vi "MOSES_v8.vi"(7 "Scan List (empty)":string="101:132,201:222", 8 "error in (no error)":errorcluster, 9 "Range (5:Auto)":T3(ring)=enum."Auto", 10 "Resolution (5:Default)":T2(ring)=enum."Default", 11 "VISA resource name":refnum<visa-resource-name>="GPIB0::9::INSTR") -> (0 "error out":errorcluster, 2 "Output Array":dbl[](array[numeric]) format="%.2f", 3 "VISA resource name out":refnum<visa-resource-name>)   [LabVIEW 2013]
doc: "This VI allows you to take simple voltage measurements from the instrument."
uses:
  Instance          12 13Saved   MOSES .vi
  Instance          62 13Saved   MOSES .vi
  Instance          11 13Saved   MOSES .vi
  Instance          63 13Saved   MOSES .vi
  Instance           9 13Saved   MOSES .vi
  Instance          64 13Saved   MOSES .vi
  Instance          10 13Saved   MOSES .vi
  Instance          60 13Saved   MOSES .vi
  Instance           8 13Saved   MOSES .vi
  Instance          33 13Saved   MOSES .vi
  Instance          75 13Saved   MOSES .vi
  Instance          37 13Saved   MOSES .vi
  Instance           5 13Saved   MOSES .vi
  Instance          32 13Saved   MOSES .vi
  Instance          74 13Saved   MOSES .vi
  Instance          38 13Saved   MOSES .vi
  Instance          72 13Saved   MOSES .vi
  Instance          41 13Saved   MOSES .vi
  Instance          71 13Saved   MOSES .vi
  Instance          40 13Saved   MOSES .vi
  Instance          73 13Saved   MOSES .vi
  Instance          39 13Saved   MOSES .vi
  Instance           6 13Saved   MOSES .vi
  Instance          35 13Saved   MOSES .vi
  Instance           7 13Saved   MOSES .vi
  Instance           4 13Saved   MOSES .vi
  Instance          34 13Saved   MOSES .vi
  Instance          16 13Saved   MOSES .vi
  Instance          52 13Saved   MOSES .vi
  Instance          17 13Saved   MOSES .vi
  Instance          58 13Saved   MOSES .vi
  Instance           1 13Saved   MOSES .vi
  Instance          53 13Saved   MOSES .vi
  Instance          15 13Saved   MOSES .vi
  Instance          59 13Saved   MOSES .vi
  Instance          19 13Saved   MOSES .vi
  Instance          57 13Saved   MOSES .vi
  Instance          18 13Saved   MOSES .vi
  Instance          56 13Saved   MOSES .vi
  Instance          20 13Saved   MOSES .vi
  Instance          55 13Saved   MOSES .vi
  Instance          22 13Saved   MOSES .vi
  Instance          54 13Saved   MOSES .vi
  Instance          21 13Saved   MOSES .vi
  Instance          51 13Saved   MOSES .vi
  Instance           2 13Saved   MOSES .vi
  Instance          50 13Saved   MOSES .vi
  Instance          23 13Saved   MOSES .vi
  Instance          49 13Saved   MOSES .vi
  Instance          24 13Saved   MOSES .vi
  Instance          48 13Saved   MOSES .vi
  Instance          26 13Saved   MOSES .vi
  Instance          47 13Saved   MOSES .vi
  Instance           3 13Saved   MOSES .vi
  Instance          70 13Saved   MOSES .vi
  Instance          27 13Saved   MOSES .vi
  Instance          66 13Saved   MOSES .vi
  Instance          25 13Saved   MOSES .vi
  Instance          69 13Saved   MOSES .vi
  Instance          28 13Saved   MOSES .vi
  Instance          68 13Saved   MOSES .vi
  Instance          30 13Saved   MOSES .vi
  Instance          67 13Saved   MOSES .vi
  Instance          31 13Saved   MOSES .vi
  Instance          45 13Saved   MOSES .vi
  Instance          29 13Saved   MOSES .vi
  Instance          44 13Saved   MOSES .vi
  Instance          65 13Saved   MOSES .vi
  Instance          43 13Saved   MOSES .vi
  Instance          46 13Saved   MOSES .vi
  Instance          42 13Saved   MOSES .vi
  Instance          36 13Saved   MOSES .vi
  Instance          13 13Saved   MOSES .vi
  Instance          14 13Saved   MOSES .vi
  Instance          61 13Saved   MOSES .vi
panel:
  in  "?":T1(tab)
  out "TEC L -y":dbl
  out "Battery":dbl
  out "Boolean 10":bool
  out "Boolean 11":bool
  out "Boolean 12":bool
  out "Mains from IS":dbl
  out "Boolean 13":bool
  out "Boolean 14":bool
  out "Boolean 15":bool
  out "12d+, MTR2812D Out":dbl
  out "Boolean 16":bool
  out "Boolean 17":bool
  out "5s, MGA2805S Out":dbl
  out "Boolean 26":bool
  out "Boolean 27":bool
  out "IS Out":dbl
  out "Boolean 20":bool
  out "Boolean 21":bool
  out "Boolean 22":bool
  out "12d+ MTR2812D Out":dbl
  out "Boolean 23":bool
  out "Boolean 24":bool
  out "Boolean 25":bool
  out "5s MGA2805S Out":dbl
  out "Boolean 29":bool
  out "Boolean 30":bool
  out "Boolean 31":bool
  out "Power Supply Filter Input":dbl
  out "Boolean 67":bool
  out "Boolean 68":bool
  out "Boolean 90":bool
  out "Boolean 7":bool
  out "Boolean 8":bool
  out "TEC L +y":dbl
  out "Boolean 6":bool
  out "Boolean 5":bool
  out "TEC L 0y":dbl
  out "Boolean 9":bool
  out "Boolean 18":bool
  out "TEC R +y":dbl
  out "Boolean 19":bool
  out "Boolean 45":bool
  out "TEC R -y":dbl
  out "Boolean 46":bool
  out "Boolean 75":bool
  out "TEC R 0y":dbl
  out "Boolean 76":bool
  out "Boolean 89":bool
  out "Thermal 5V power":dbl
  out "Shutter 28V power":dbl
  out "H-alpha filter":dbl
  out "H-alpha camera":dbl
  out "ROE power supply input":dbl
  out "Premod filter positive 12V input":dbl
  out "Premod filter 5V input":dbl
  out "Shutter 28V power":dbl
  out "H-alpha filter":dbl
  out "ROE power supply input":dbl
  out "Boolean 41":bool
  out "Boolean 42":bool
  out "Res +y":dbl
  out "Res -y":dbl
  out "Res Back":dbl
  out "Boolean 43":bool
  out "Boolean 44":bool
  out "Boolean 47":bool
  out "Boolean 48":bool
  out "Boolean 49":bool
  out "Boolean 50":bool
  out "CF +y":dbl
  out "CF -y":dbl
  out "CF 0y":dbl
  out "Boolean 51":bool
  out "Boolean 52":bool
  out "Boolean 53":bool
  out "Boolean 54":bool
  out "BP +y":dbl
  out "BP -y":dbl
  out "BP 0y":dbl
  out "Boolean 55":bool
  out "Boolean 56":bool
  out "Boolean 57":bool
  out "Boolean 58":bool
  out "Boolean 59":bool
  out "Boolean 60":bool
  out "Boolean 40":bool
  out "PCU Res":dbl
  out "Boolean 83":bool
  out "Boolean 84":bool
  out "ICU":dbl
  out "Boolean 85":bool
  out "Boolean 86":bool
  out "PCU Box":dbl
  out "Boolean 87":bool
  out "Boolean 88":bool
  out "Boolean 32":bool
  out "Boolean 33":bool
  out "Boolean 34":bool
  out "TEC +y":dbl
  out "TEC -y":dbl
  out "TEC 0y":dbl
  out "Boolean 35":bool
  out "Boolean 36":bool
  out "Boolean 37":bool
  out "Boolean 38":bool
  out "Boolean 39":bool
  out "Comp Res":dbl
  out "Boolean 61":bool
  out "Boolean 62":bool
  out "Vortec x86 CPU":dbl
  out "Boolean 63":bool
  out "Boolean 64":bool
  out "Mainboard":dbl
  out "Boolean 65":bool
  out "Boolean 66":bool
  out "Virtex 5 FPGA":dbl
  out "Boolean 69":bool
  out "Boolean 70":bool
  out "RPA":dbl
  out "Boolean 71":bool
  out "Boolean 72":bool
  out "TC Res.":dbl
  out "Boolean 73":bool
  out "Boolean 74":bool
  out "T CONT b -y":dbl
  out "Boolean 77":bool
  out "Boolean 78":bool
  out "12S":dbl
  out "Boolean 79":bool
  out "Boolean 80":bool
  out "12D":dbl
  out "Boolean 81":bool
  out "Boolean 82":bool
  out "0 Order TECs":dbl[][](graph)
  out "-1 Order TECs":dbl[][](graph)
  out "+1 Order TECs":dbl[][](graph)
  out "I5s":dbl[](graph)
  out "I12d+":dbl[](graph)
  out "Iout":dbl[](graph)
  out "Power Supply Filter Input":dbl[](graph)
  out "TEC Currents":dbl[][](graph)
  out "Back Plates":dbl[][](graph)
  out "Cold Fingers":dbl[][](graph)
  out "CONT":dbl[][](graph)
  out "PCU":dbl[][](graph)
  out "COMP":dbl[][](graph)
  out "Reservoir":dbl[][](graph)
  out "ROE":dbl[](graph)
  out "PSU":dbl[](graph)
  in  "C":dbl
  in  "B":dbl
  in  "A":dbl
  in  "stop 2":bool
  # "System"
  # "System"
  # "Voltage"
  # "Current"
  # "C"
  # "V"
  # "A"
  # "Temperatures of \n+1 Order CCD\nThermal Reservoir, Cold Finger, and Back Plate"
  # "C"
  # "A"
  # "V"
  # "C"
  # "A"
  # "V"
  # "Temperatures of \n0 Order CCD\nCold Finger and Back Plate"
  # "C"
  # "V"
  # "mA"
  # "C"
  # "Thermo Electric Coolers (TEC)"
  # "CCD"
  # "Voltage on L or R side of TEC"
  # "Current"
  # "C"
  # "Temperatures of \n-1 Order CCD\nThermal Reservoir, Cold Finger, and Back Plate"
  # "V"
  # "C"
  # "+1 Order"
  # "A"
  # "V"
  # "C"
  # "Temperature of\nBack of Thermal Reservoir"
  # "C"
  # "V"
  # "0 Order"
  # "A"
  # "Computer"
  # "V"
  # "C"
  # "C"
  # "C"
  # "V"
  # "-1 Order"
  # "A"
  # "C"
  # "C"
  # "C"
  # "V"
  # "Sub-Systems"
  # "C"
  # "C"
  # "Current"
  # "Voltage"
  # "C"
  # "C"
  # "mA"
  # "V"
  # "C"
  # "C"
  # "V"
  # "mA"
  # "V"
  # "A"
  # "V"
  # "A"
  # "V"
  # "A"
  # "Please add graphs and values that you would like to see in the text box below."
  # "Flight Screen:\n-TECs\n-\n-"
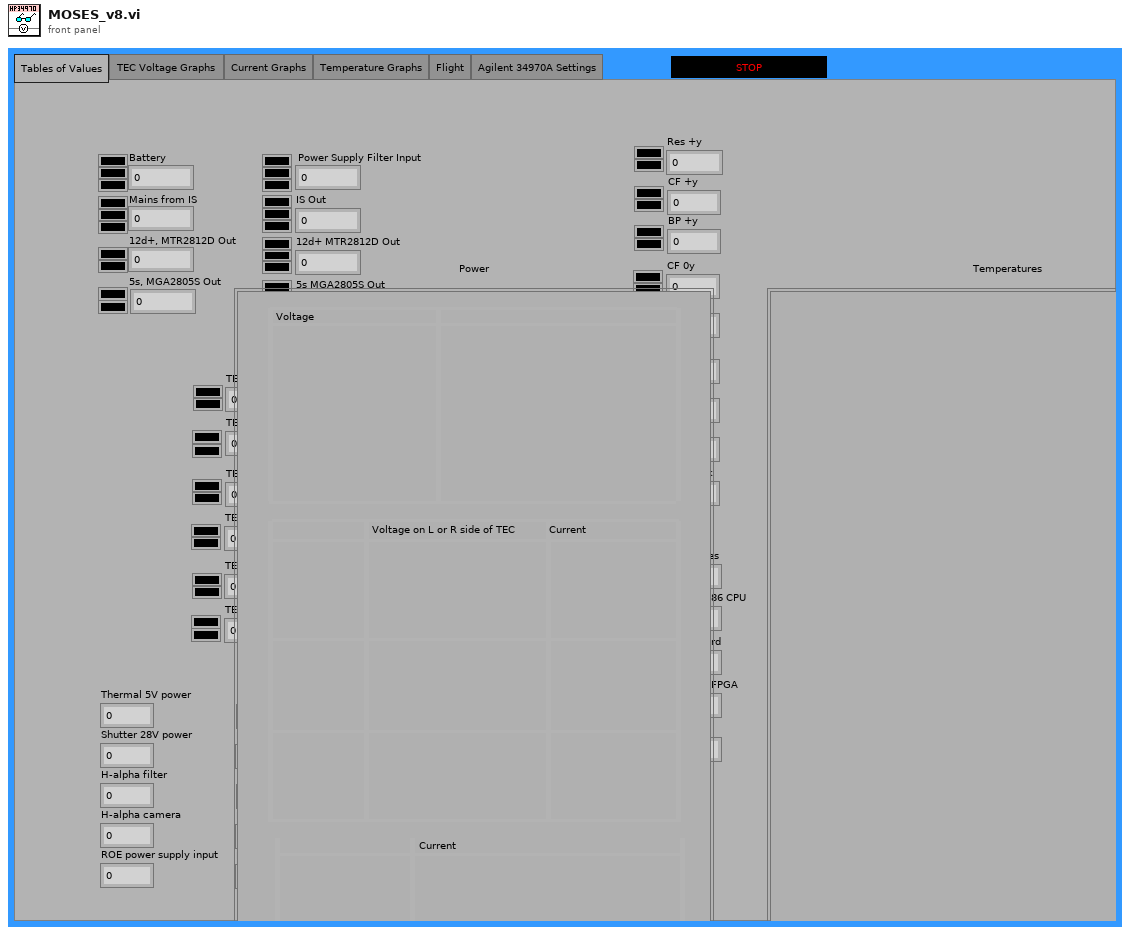
[diagram p1: front panel]
types:
  T1 = enum32{"Tables of Values", "TEC Voltage Graphs ", "Current Graphs", "Temperature Graphs", "Flight", "Agilent 34970A Settings"}
  T2 = enum16{"4 1/2", "5 1/2", "6 1/2", "Least", "Highest", "Default"}
  T3 = enum16{"100 mV", "1 V", "10 V", "100 V", "300 V", "Auto", "Minimum", "Maximum"}
  T4 = cluster{"Output Number Array[0]":dbl, "Output Number Array[1]":dbl, "Output Number Array[2]":dbl, "Output Number Array[3]":dbl, "Output Number Array[4]":dbl, "Output Number Array[5]":dbl, "Output Number Array[6]":dbl, "Output Number Array[7]":dbl, "Output Number Array[8]":dbl, "Output Number Array[9]":dbl, "Output Number Array[10]":dbl, "Output Number Array[11]":dbl, "Output Number Array[12]":dbl, "Output Number Array[13]":dbl, "Output Number Array[14]":dbl, "Output Number Array[15]":dbl, "Output Number Array[16]":dbl, "Output Number Array[17]":dbl, "Output Number Array[18]":dbl, "Output Number Array[19]":dbl, "Output Number Array[20]":dbl, "Output Number Array[21]":dbl, "Output Number Array[22]":dbl, "Output Number Array[23]":dbl, "Output Number Array[24]":dbl, "Output Number Array[25]":dbl, "Output Number Array[26]":dbl, "Output Number Array[27]":dbl, "Output Number Array[28]":dbl, "Output Number Array[29]":dbl, "Output Number Array[30]":dbl, "Output Number Array[31]":dbl, "Output Number Array[32]":dbl, "Output Number Array[33]":dbl, "Output Number Array[34]":dbl, "Output Number Array[35]":dbl, "Output Number Array[36]":dbl, "Output Number Array[37]":dbl, "Output Number Array[38]":dbl, "Output Number Array[39]":dbl, "Output Number Array[40]":dbl, "Output Number Array[41]":dbl, "Output Number Array[42]":dbl, "Output Number Array[43]":dbl, "Output Number Array[44]":dbl, "Output Number Array[45]":dbl, "Output Number Array[46]":dbl, "Output Number Array[47]":dbl, "Output Number Array[48]":dbl, "Output Number Array[49]":dbl, "Output Number Array[50]":dbl, "Output Number Array[51]":dbl, "Output Number Array[52]":dbl, "Output Number Array[53]":dbl, "Output Number Array[54]":dbl, "Output Number Array[55]":dbl, "Output Number Array[56]":dbl, "Output Number Array[57]":dbl, "Output Number Array[58]":dbl, "Output Number Array[59]":dbl, "Output Number Array[60]":dbl, "Output Number Array[61]":dbl, "Output Number Array[62]":dbl, "Output Number Array[63]":dbl, "Output Number Array[64]":dbl, "Output Number Array[65]":dbl, "Output Number Array[66]":dbl, "Output Number Array[67]":dbl, "Output Number Array[68]":dbl, "Output Number Array[69]":dbl}
  T5 = cluster{"V5s, MGA2805S output voltage":dbl, "T5V, Thermal 5V power voltage":dbl, "S28V, Shutter 28V power voltage":dbl, "HAFV, H-alpha filter voltage":dbl, "HACV, H-alpha camera voltage":dbl, "If_in, Power supply filter input current":dbl, "Ipf12+, Premod filter positive 12V input current":dbl, "I_pf5, Premod filter 5V input current":dbl, "S28I, Shutter 28V power current":dbl, "HAFI, H-alpha filter current":dbl, "ROE_PSV, ROE power supply input voltage":dbl, "ROE_PSI, ROE power supply input current":dbl, "T_ROE, ROE Temp.":dbl, "T_PSU, PSU Temp.":dbl}
diagram:
  # "This goes to MOSES background."
  n1 = while {
    shift-right: [w661] -> _
    shift-left: _ -> [w662]
    shift-right: [w652] -> w4
    shift-left: _ -> [w653]
    shift-right: [w650] -> _
    shift-left: _ -> [w651]
    shift-right: [w634] -> w5
    shift-left: _ -> [w635]
    shift-right: [w631] -> w6
    shift-left: _ -> [w632]
    shift-right: [w438] -> w16
    shift-left: _ -> [w610]
    shift-right: [w437] -> w15
    shift-left: _ -> [w606]
    shift-right: [w436] -> w14
    shift-left: _ -> [w186]
    shift-right: [w591] -> w13
    shift-left: _ -> [w593]
    shift-right: [w562] -> w7
    shift-left: _ -> [w575]
    shift-right: [w148] -> w12
    shift-left: _ -> [w543]
    shift-right: [w363] -> w11
    shift-left: _ -> [w522]
    shift-right: [w516] -> _
    shift-left: _ -> [w517]
    shift-right: [w474] -> _
    shift-left: _ -> [w473]
    shift-right: [w472] -> _
    shift-left: _ -> [w471]
    shift-right: [w468] -> _
    shift-left: _ -> [w469]
    shift-right: [w467] -> _
    shift-left: _ -> [w466]
    shift-right: [w465] -> _
    shift-left: _ -> [w464]
    shift-right: [w463] -> _
    shift-left: _ -> [w462]
    shift-right: [w461] -> _
    shift-left: _ -> [w460]
    shift-right: [w459] -> _
    shift-left: _ -> [w187]
    shift-right: [w458] -> _
    shift-left: _ -> [w457]
    shift-right: [w456] -> _
    shift-left: _ -> [w455]
    shift-right: [w454] -> _
    shift-left: _ -> [w453]
    shift-right: [w66] -> _
    shift-left: _ -> [w180]
    shift-right: [w445] -> _
    shift-left: _ -> [w444]
    shift-right: [w92] -> _
    shift-left: _ -> [w446]
    shift-right: [w443] -> _
    shift-left: _ -> [w442]
    shift-right: [w441] -> _
    shift-left: _ -> [w440]
    shift-right: [w362] -> w8
    shift-left: _ -> [w376]
    shift-right: [w374] -> _
    shift-left: _ -> [w375]
    shift-right: [w373] -> _
    shift-left: _ -> [w372]
    shift-right: [w371] -> _
    shift-left: _ -> [w370]
    shift-right: [w368] -> _
    shift-left: _ -> [w369]
    shift-right: [w364] -> _
    shift-left: _ -> [w365]
    shift-right: [w367] -> _
    shift-left: _ -> [w366]
    shift-right: [w312] -> w10
    shift-left: _ -> [w322]
    shift-right: [w320] -> _
    shift-left: _ -> [w319]
    shift-right: [w318] -> _
    shift-left: _ -> [w317]
    shift-right: [w315] -> _
    shift-left: _ -> [w316]
    shift-right: [w314] -> _
    shift-left: _ -> [w313]
    shift-right: [w278] -> _
    shift-left: _ -> [w279]
    shift-right: [w277] -> _
    shift-left: _ -> [w276]
    shift-right: [w274] -> _
    shift-left: _ -> [w275]
    shift-right: [w273] -> w9
    shift-left: _ -> [w280]
    stop <- "stop 2" stop-if-true
    w78 = 0.05 ("y")
    w79 = 4.0 ("y")
    w84 = 2.5 ("y")
    w122 = 2.5 ("y")
    w126 = 2.5 ("y")
    w130 = 2.5 ("y")
    w133 = 2.5 ("y")
    (unwired) 37482.0 ("double precision float")
    (unwired) 9360000.0 ("double precision float")
    (unwired) 9.3e-08 ("double precision float")
    (unwired) 0.000236053 ("double precision float")
    (unwired) 9.3e-08 ("double precision float")
    (unwired) 0.000236053 ("double precision float")
    (unwired) 0.001285847 ("double precision float")
    (unwired) 0.001285847 ("double precision float")
    w72 = 150.0 ("y")
    w76 = 300.0 ("y")
    w107 = 2.5 ("y")
    w25 = 0.03 ("y")
    w112 = 3.0 ("y")
    w32 = 0.01 ("y")
    w655 = 2.5 ("y")
    w657 = 2.5 ("y")
    # "File saves to data.txt on the desktop."
    # "These four need real equations and alarm limits."
    # "For highest resolution\nmeasurements, \nchange VISA timeout"
    n2 = Append True/False String(1:FALSE ("selector"), 2:"DC? ", 3:"AC? ", 4:"MEAS:VOLT:") -> (0:w669:string)
    n3 = Pick Line(string ("")=w669, multi-line string=".1,\n1,\n10,\n100,\n300,\nAUTO\nMIN,\nMAX,", line index="Range (5:Auto)") -> (output string=w666:string)
    n4 = case shown="Default" "Range (5:Auto)" {
      selector: "Range (5:Auto)" -> [_ w695]
      tunnel: [w689 w692] -> w665
      tunnel: w666 -> [w689 w691]
      tunnel: "Resolution (5:Default)" -> [_ w693]
      frame "Auto" {
        # "Autorange"
      }
      frame Default {
        # "Not Autorange"
        n5 = Index Array(array=dbl[] [0.1, 1.0, 10.0, 100.0, 300.0, 0.0, 0.1, 300.0], index=w695) -> (element=w690:dbl)
        n6 = case shown="Default" w693 {
          selector: w693 -> [w702 _ _ _]
          tunnel: [w696 w706 w709 w710] -> w692
          tunnel: w691 -> [w699 w705 w707 w711]
          tunnel: w690 -> [w701 _ _ _]
          frame Default {
            # "4.5, 5.5, or 6.5 Digits *"
            n7 = Index Array(array=dbl[] [0.0001, 3e-06, 1e-06], index=w702) -> (element=w700:dbl)
            n8 = Multiply(x=w700, y=w701) -> (x*y=w698:dbl)
            n9 = Format Into String(format string="%.; %e", initial string=w699, w698) -> (resulting string=w696:string)  [unwired: 1 in, 1 out]
          }
          frame "Least" {
            # "Least resolution"
            n10 = Concatenate Strings(w705, " MAX" ("string")) -> (w706:string)
          }
          frame "Highest" {
            # "Highest range"
            n11 = Concatenate Strings(w707, " MIN" ("string")) -> (w709:string)
          }
          frame "Default" {
            # "Default range"
            n12 = Concatenate Strings(w711, " DEF" ("string")) -> (w710:string)
          }
        }
      }
    }
    n13 = call "Convert to Dynamic Data3"() -> ("Dynamic Data Type"=w589:dynamicdata)  [unwired: 4 in]
    n14 = call "Formula10"("V1"=5000, "28V"=w589, "R1"=28) -> ("Result"=w584:dynamicdata)  [unwired: 11 in, 1 out]
    n15 = Concatenate Strings(w665, ", (@", "Scan List (empty)", ")") -> (w676:string)
    n16 = VISA Write(VISA resource name="VISA resource name", write buffer=w676, error in (no error)="error in (no error)") -> (VISA resource name out=w685:refnum<visa-resource-name>, error out=w684:errorcluster)  [unwired: 1 out]
    n17 = call "Formula9"("X1"=5000, "X2"=5000, "X3"=5000, "X4"=w584) -> ("Result"=w590:dynamicdata)  [unwired: 10 in, 1 out]
    n18 = property class="Instr"(reference=w685, error in=w684, "General Settings:Timeout Value"=u32 320000 ("Tmo Value")) -> (reference out=w682:refnum<visa-resource-name>, error out=w683:errorcluster)
    n19 = call "Convert from Dynamic Data9"("Dynamic Data Type"=w590) -> ()  [unwired: 3 in, 1 out]
    n20 = Get Date/Time String(want seconds? (F)=TRUE) -> (time string=w664:string)  [unwired: 2 in, 1 out]
    n21 = VISA Read(VISA resource name=w682, byte count=u32 4088 ("byte count (0)"), error in (no error)=w683) -> (VISA resource name out=→"VISA resource name out":refnum<visa-resource-name>, read buffer=w677:string, error out=→"error out":errorcluster)  [unwired: 1 out]
    n22 = call <instrlib>:"HP34970A List to Array.vi"("List (empty)"=w677) -> ("Output Number Array"=w185:dbl[])  [unwired: 5 in, 1 out]
    "Output Array" <- w185
    n23 = call "sub_vi.vi"("Array"=w185) -> ("Dynamic Data Type"=w659:dynamicdata)  [unwired: 3 in]
    n24 = call "Write LabVIEW Measurement File2"("Comment"=w664, "Signals"=w659) -> ()  [unwired: 7 in, 3 out]
    n25 = Array To Cluster(array=w185) -> (cluster=w654:T4)
    n26 = Build Array (concatenate)(w662, w185) -> (w661:dbl[][])
    n27 = Unbundle(w654) -> ("Output Number Array[0]"=w137:dbl, "Output Number Array[1]"=w23:dbl, "Output Number Array[2]"=w135:dbl, "Output Number Array[3]"=w129:dbl, "Output Number Array[4]"=w125:dbl, "Output Number Array[5]"=w121:dbl, "Output Number Array[8]"=w143:dbl, "Output Number Array[9]"=w146:dbl, "Output Number Array[10]"=w150:dbl, "Output Number Array[11]"=w101:dbl, "Output Number Array[16]"=w179:dbl, "Output Number Array[17]"=w91:dbl, "Output Number Array[18]"=w178:dbl, "Output Number Array[19]"=w177:dbl, "Output Number Array[22]"=w176:dbl, "Output Number Array[23]"=w175:dbl, "Output Number Array[24]"=w174:dbl, "Output Number Array[29]"=w173:dbl, "Output Number Array[30]"=w172:dbl, "Output Number Array[32]"=w171:dbl, "Output Number Array[33]"=w170:dbl, "Output Number Array[34]"=w169:dbl, "Output Number Array[35]"=w168:dbl, "Output Number Array[36]"=w167:dbl, "Output Number Array[37]"=w166:dbl, "Output Number Array[38]"=w165:dbl, "Output Number Array[39]"=w164:dbl, "Output Number Array[40]"=w163:dbl, "Output Number Array[41]"=w162:dbl, "Output Number Array[42]"=w161:dbl, "Output Number Array[43]"=w160:dbl, "Output Number Array[44]"=w159:dbl, "Output Number Array[45]"=w158:dbl, "Output Number Array[46]"=w151:dbl, "Output Number Array[49]"=w155:dbl, "Output Number Array[50]"=w156:dbl, "Output Number Array[51]"=w154:dbl, "Output Number Array[52]"=w152:dbl, "Output Number Array[53]"=w153:dbl)  [unwired: 31 out]
    "TEC L +y" <- w137
    "TEC L 0y" <- w135
    "TEC R +y" <- w129
    "TEC R -y" <- w125
    "TEC R 0y" <- w121
    "TEC L -y" <- w23
    n28 = call "Formula6"("X1"=w176) -> ("Result"=w596:dynamicdata)  [unwired: 13 in, 1 out]
    n29 = call "Formula11"("a"=0.001285847 ("double precision float"), "v0"=w173, "b"=0.000236053 ("double precision float"), "c"=9.3e-08 ("double precision float"), "R"=9360000.0 ("double precision float")) -> ("Result"=w578:dynamicdata)  [unwired: 9 in, 1 out]
    n30 = call "Formula13"("a"=0.001285847 ("double precision float"), "v0"=w171, "b"=0.000236053 ("double precision float"), "c"=9.3e-08 ("double precision float"), "R"=9360000.0 ("double precision float")) -> ("Result"=w563:dynamicdata)  [unwired: 9 in, 1 out]
    n31 = call "Formula14"("a"=0.001285847 ("double precision float"), "v0"=w170, "b"=0.000236053 ("double precision float"), "c"=9.3e-08 ("double precision float"), "R"=1420000.0 ("double precision float")) -> ("Result"=w556:dynamicdata)  [unwired: 9 in, 1 out]
    n32 = call "Formula18"("a"=0.001285847 ("double precision float"), "v0"=w166, "b"=0.000236053 ("double precision float"), "c"=9.3e-08 ("double precision float"), "R"=1420000.0 ("double precision float")) -> ("Result"=w530:dynamicdata)  [unwired: 9 in, 1 out]
    n33 = call "Formula29"("a"=0.001285847 ("double precision float"), "v0"=w153, "b"=0.000236053 ("double precision float"), "c"=9.3e-08 ("double precision float"), "R"=37482.0 ("double precision float")) -> ("Result"=w329:dynamicdata)  [unwired: 9 in, 1 out]
    n34 = call "Formula32"("a"=0.001285847 ("double precision float"), "v0"=w156, "b"=0.000236053 ("double precision float"), "c"=9.3e-08 ("double precision float"), "R"=37482.0 ("double precision float")) -> ("Result"=w288:dynamicdata)  [unwired: 9 in, 1 out]
    n35 = call "Formula7"("X1"=w175) -> ("Result"=w595:dynamicdata)  [unwired: 13 in, 1 out]
    n36 = call "Formula8"("X1"=w174) -> ("Result"=w594:dynamicdata)  [unwired: 13 in, 1 out]
    n37 = call "Formula16"("a"=0.001285847 ("double precision float"), "v0"=w168, "b"=0.000236053 ("double precision float"), "c"=9.3e-08 ("double precision float"), "R"=1420000.0 ("double precision float")) -> ("Result"=w544:dynamicdata)  [unwired: 9 in, 1 out]
    n38 = call "Formula28"("a"=0.001285847 ("double precision float"), "v0"=w152, "b"=0.000236053 ("double precision float"), "c"=9.3e-08 ("double precision float"), "R"=37482.0 ("double precision float")) -> ("Result"=w338:dynamicdata)  [unwired: 9 in, 1 out]
    n39 = call "Formula31"("a"=0.001285847 ("double precision float"), "v0"=w154, "b"=0.000236053 ("double precision float"), "c"=9.3e-08 ("double precision float"), "R"=37482.0 ("double precision float")) -> ("Result"=w297:dynamicdata)  [unwired: 9 in, 1 out]
    n40 = call "Formula12"("a"=0.001285847 ("double precision float"), "v0"=w172, "b"=0.000236053 ("double precision float"), "c"=9.3e-08 ("double precision float"), "R"=9360000.0 ("double precision float")) -> ("Result"=w569:dynamicdata)  [unwired: 9 in, 1 out]
    n41 = call "Formula17"("a"=0.001285847 ("double precision float"), "v0"=w167, "b"=0.000236053 ("double precision float"), "c"=9.3e-08 ("double precision float"), "R"=1420000.0 ("double precision float")) -> ("Result"=w536:dynamicdata)  [unwired: 9 in, 1 out]
    n42 = call "Formula19"("a"=0.001285847 ("double precision float"), "v0"=w165, "b"=0.000236053 ("double precision float"), "c"=9.3e-08 ("double precision float"), "R"=1420000.0 ("double precision float")) -> ("Result"=w524:dynamicdata)  [unwired: 9 in, 1 out]
    n43 = call "Formula22"("a"=0.001285847 ("double precision float"), "v0"=w162, "b"=0.000236053 ("double precision float"), "c"=9.3e-08 ("double precision float"), "R"=37482.0 ("double precision float")) -> ("Result"=w412:dynamicdata)  [unwired: 9 in, 1 out]
    n44 = call "Formula23"("a"=0.001285847 ("double precision float"), "v0"=w161, "b"=0.000236053 ("double precision float"), "c"=9.3e-08 ("double precision float"), "R"=37482.0 ("double precision float")) -> ("Result"=w404:dynamicdata)  [unwired: 9 in, 1 out]
    n45 = call "Formula26"("a"=0.001285847 ("double precision float"), "v0"=w158, "b"=0.000236053 ("double precision float"), "c"=9.3e-08 ("double precision float"), "R"=37482.0 ("double precision float")) -> ("Result"=w356:dynamicdata)  [unwired: 9 in, 1 out]
    n46 = call "Formula30"("a"=0.001285847 ("double precision float"), "v0"=w155, "b"=0.000236053 ("double precision float"), "c"=9.3e-08 ("double precision float"), "R"=37482.0 ("double precision float")) -> ("Result"=w306:dynamicdata)  [unwired: 9 in, 1 out]
    n47 = call "Formula15"("a"=0.001285847 ("double precision float"), "v0"=w169, "b"=0.000236053 ("double precision float"), "c"=9.3e-08 ("double precision float"), "R"=1420000.0 ("double precision float")) -> ("Result"=w550:dynamicdata)  [unwired: 9 in, 1 out]
    n48 = call "Formula20"("a"=0.001285847 ("double precision float"), "v0"=w164, "b"=0.000236053 ("double precision float"), "c"=9.3e-08 ("double precision float"), "R"=291400.0 ("double precision float")) -> ("Result"=w430:dynamicdata)  [unwired: 9 in, 1 out]
    n49 = call "Formula25"("a"=0.001285847 ("double precision float"), "v0"=w159, "b"=0.000236053 ("double precision float"), "c"=9.3e-08 ("double precision float"), "R"=37482.0 ("double precision float")) -> ("Result"=w386:dynamicdata)  [unwired: 9 in, 1 out]
    n50 = call "Formula21"("a"=0.001285847 ("double precision float"), "v0"=w163, "b"=0.000236053 ("double precision float"), "c"=9.3e-08 ("double precision float"), "R"=37482.0 ("double precision float")) -> ("Result"=w421:dynamicdata)  [unwired: 9 in, 1 out]
    n51 = call "Formula24"("a"=0.001285847 ("double precision float"), "v0"=w160, "b"=0.000236053 ("double precision float"), "c"=9.3e-08 ("double precision float"), "R"=37482.0 ("double precision float")) -> ("Result"=w395:dynamicdata)  [unwired: 9 in, 1 out]
    n52 = call "Formula27"("a"=0.001285847 ("double precision float"), "v0"=w151, "b"=0.000236053 ("double precision float"), "c"=9.3e-08 ("double precision float"), "R"=37482.0 ("double precision float")) -> ("Result"=w347:dynamicdata)  [unwired: 9 in, 1 out]
    n53 = call "Formula4"("X1"=w178) -> ("Result"=w607:dynamicdata)  [unwired: 13 in, 1 out]
    n54 = call "Formula37"("X1"=w91) -> ("Result"=w93:dynamicdata)  [unwired: 13 in, 1 out]
    n55 = call "Formula3"("X1"=w179) -> ("Result"=w611:dynamicdata)  [unwired: 13 in, 1 out]
    n56 = call "Formula5"("X1"=w177) -> ("Result"=w602:dynamicdata)  [unwired: 13 in, 1 out]
    n57 = call "Formula34"("X1"=w146) -> ("Result"=w145:dynamicdata)  [unwired: 13 in, 1 out]
    n58 = call "Formula33"("X1"=w150) -> ("Result"=w149:dynamicdata)  [unwired: 13 in, 1 out]
    n59 = call "Formula35"("X1"=w143) -> ("Result"=w144:dynamicdata)  [unwired: 13 in, 1 out]
    n60 = call "Formula36"("X1"=w101) -> ("Result"=w102:dynamicdata)  [unwired: 13 in, 1 out]
    n61 = call "Convert from Dynamic Data11"("Dynamic Data Type"=w569) -> ("Scalar"=w17:dbl)  [unwired: 3 in]
    "Res -y" <- w17
    n62 = call "Convert from Dynamic Data32"("Dynamic Data Type"=w297) -> ("Scalar"=w283:dbl)  [unwired: 3 in]
    "ICU" <- w283
    n63 = call "Convert from Dynamic Data33"("Dynamic Data Type"=w288) -> ("Scalar"=w282:dbl)  [unwired: 3 in]
    "PCU Box" <- w282
    n64 = call "Convert from Dynamic Data7"("Dynamic Data Type"=w595) -> ("Scalar"=w51:dbl)  [unwired: 3 in]
    "TEC -y" <- w51
    n65 = call "Convert from Dynamic Data8"("Dynamic Data Type"=w594) -> ("Scalar"=w40:dbl)  [unwired: 3 in]
    "TEC 0y" <- w40
    n66 = call "Convert from Dynamic Data10"("Dynamic Data Type"=w578) -> ("Scalar"=w577:dbl)  [unwired: 3 in]
    "Res +y" <- w577
    n67 = call "Convert from Dynamic Data13"("Dynamic Data Type"=w563) -> ("Scalar"=w18:dbl)  [unwired: 3 in]
    "Res Back" <- w18
    n68 = call "Convert from Dynamic Data14"("Dynamic Data Type"=w556) -> ("Scalar"=w542:dbl)  [unwired: 3 in]
    "CF +y" <- w542
    n69 = call "Convert from Dynamic Data29"("Dynamic Data Type"=w338) -> ("Scalar"=w324:dbl)  [unwired: 3 in]
    "12S" <- w324
    n70 = call "Convert from Dynamic Data30"("Dynamic Data Type"=w329) -> ("Scalar"=w323:dbl)  [unwired: 3 in]
    "12D" <- w323
    n71 = call "Convert from Dynamic Data6"("Dynamic Data Type"=w596) -> ("Scalar"=w67:dbl)  [unwired: 3 in]
    "TEC +y" <- w67
    n72 = call "Convert from Dynamic Data15"("Dynamic Data Type"=w550) -> ("Scalar"=w21:dbl)  [unwired: 3 in]
    "CF -y" <- w21
    n73 = call "Convert from Dynamic Data16"("Dynamic Data Type"=w544) -> ("Scalar"=w22:dbl)  [unwired: 3 in]
    "CF 0y" <- w22
    n74 = call "Convert from Dynamic Data17"("Dynamic Data Type"=w536) -> ("Scalar"=w521:dbl)  [unwired: 3 in]
    "BP +y" <- w521
    n75 = call "Convert from Dynamic Data18"("Dynamic Data Type"=w530) -> ("Scalar"=w19:dbl)  [unwired: 3 in]
    "BP -y" <- w19
    n76 = call "Convert from Dynamic Data19"("Dynamic Data Type"=w524) -> ("Scalar"=w20:dbl)  [unwired: 3 in]
    "BP 0y" <- w20
    n77 = call "Convert from Dynamic Data28"("Dynamic Data Type"=w347) -> ("Scalar"=w157:dbl)  [unwired: 3 in]
    "T CONT b -y" <- w157
    n78 = call "Convert from Dynamic Data31"("Dynamic Data Type"=w306) -> ("Scalar"=w284:dbl)  [unwired: 3 in]
    "PCU Res" <- w284
    n79 = call "Convert from Dynamic Data5"("Dynamic Data Type"=w602) -> ("Scalar"=w73:dbl)  [unwired: 3 in]
    "5s MGA2805S Out" <- w73
    n80 = call "Convert from Dynamic Data20"("Dynamic Data Type"=w430) -> ("Scalar"=w382:dbl)  [unwired: 3 in]
    "Comp Res" <- w382
    n81 = call "Convert from Dynamic Data26"("Dynamic Data Type"=w356) -> ("Scalar"=w325:dbl)  [unwired: 3 in]
    "TC Res." <- w325
    n82 = call "Convert from Dynamic Data3"("Dynamic Data Type"=w607) -> ("Scalar"=w108:dbl)  [unwired: 3 in]
    "12d+ MTR2812D Out" <- w108
    n83 = Less?(x=w108, y=w107) -> (x < y?=w24:bool)
    n84 = Absolute Value(x=w108) -> (abs(x)=w26:dbl)
    n85 = call "Convert from Dynamic Data21"("Dynamic Data Type"=w421) -> ("Scalar"=w381:dbl)  [unwired: 3 in]
    "Vortec x86 CPU" <- w381
    n86 = call "Convert from Dynamic Data22"("Dynamic Data Type"=w412) -> ("Scalar"=w380:dbl)  [unwired: 3 in]
    "Mainboard" <- w380
    n87 = call "Convert from Dynamic Data23"("Dynamic Data Type"=w404) -> ("Scalar"=w103:dbl)  [unwired: 3 in]
    n88 = call "Convert from Dynamic Data24"("Dynamic Data Type"=w395) -> ("Scalar"=w379:dbl)  [unwired: 3 in]
    "Virtex 5 FPGA" <- w379
    n89 = call "Convert from Dynamic Data25"("Dynamic Data Type"=w386) -> ("Scalar"=w378:dbl)  [unwired: 3 in]
    "RPA" <- w378
    n90 = call "Convert from Dynamic Data2"("Dynamic Data Type"=w611) -> ("Scalar"=w113:dbl)  [unwired: 3 in]
    "IS Out" <- w113
    n91 = Absolute Value(x=w113) -> (abs(x)=w33:dbl)
    n92 = Less?(x=w113, y=w112) -> (x < y?=w29:bool)
    n93 = Less?(x=w23, y=w657) -> (x < y?=→"Boolean 6":bool)
    n94 = Greater?(x=w73, y=w76) -> (0:w604:bool)
    n95 = Greater?(x=w67, y=2.85) -> (0:→"Boolean 32":bool)
    n96 = Greater?(x=w33, y=w32) -> (0:w30:bool)
    n97 = Greater?(x=w26, y=w25) -> (0:w27:bool)
    n98 = Less?(x=w17, y=-65.0) -> (x < y?=w571:bool)
    n99 = Less?(x=w283, y=0.0) -> (x < y?=w299:bool)
    n100 = Less?(x=w282, y=15.0) -> (x < y?=w290:bool)
    n101 = Less?(x=w577, y=-65.0) -> (x < y?=w580:bool)
    n102 = Less?(x=w18, y=-65.0) -> (x < y?=w565:bool)
    n103 = Less?(x=w542, y=-31.0) -> (x < y?=w558:bool)
    n104 = Less?(x=w324, y=15.0) -> (x < y?=w340:bool)
    n105 = Less?(x=w323, y=15.0) -> (x < y?=w331:bool)
    n106 = Less?(x=w21, y=-31.0) -> (x < y?=w552:bool)
    n107 = Less?(x=w22, y=-31.0) -> (x < y?=w546:bool)
    n108 = Less?(x=w521, y=-55.0) -> (x < y?=w538:bool)
    n109 = Less?(x=w19, y=-55.0) -> (x < y?=w532:bool)
    n110 = Less?(x=w20, y=-55.0) -> (x < y?=w526:bool)
    n111 = Less?(x=w157, y=15.0) -> (x < y?=w349:bool)
    n112 = Less?(x=w284, y=15.0) -> (x < y?=w308:bool)
    n113 = Greater?(x=w51, y=2.75) -> (0:→"Boolean 35":bool)
    n114 = Less?(x=w382, y=0.0) -> (x < y?=w432:bool)
    n115 = Less?(x=w325, y=15.0) -> (x < y?=w358:bool)
    n116 = Greater?(x=w40, y=2.75) -> (0:→"Boolean 38":bool)
    n117 = Less?(x=w381, y=6.0) -> (x < y?=w423:bool)
    n118 = Less?(x=w380, y=6.0) -> (x < y?=w414:bool)
    n119 = Less?(x=w103, y=10.8) -> (x < y?=w405:bool)
    n120 = Less?(x=w379, y=6.0) -> (x < y?=w397:bool)
    n121 = Less?(x=w378, y=6.0) -> (x < y?=w388:bool)
    n122 = call "Convert from Dynamic Data12"("Dynamic Data Type"=w93) -> ("Scalar"=w80:dbl)  [unwired: 3 in]
    "Power Supply Filter Input" <- w80
    n123 = call "Convert from Dynamic Data36"("Dynamic Data Type"=w145) -> ("Scalar"=w117:dbl)  [unwired: 3 in]
    "Mains from IS" <- w117
    n124 = call "Convert from Dynamic Data34"("Dynamic Data Type"=w149) -> ("Scalar"=w115:dbl)  [unwired: 3 in]
    "12d+, MTR2812D Out" <- w115
    n125 = call "Convert from Dynamic Data37"("Dynamic Data Type"=w144) -> ("Scalar"=w142:dbl)  [unwired: 3 in]
    "Battery" <- w142
    n126 = call "Convert to Dynamic Data2"("Array"=w185) -> ("Dynamic Data Type"=w647:dynamicdata)  [unwired: 3 in]
    n127 = And(x=w29, y=w30) -> (x .and. y?=w31:bool)
    "Boolean 20" <- w31
    n128 = And(x=w24, y=w27) -> (x .and. y?=w28:bool)
    "Boolean 23" <- w28
    n129 = Absolute Value(x=w142) -> (abs(x)=w640:dbl)
    n130 = Absolute Value(x=w117) -> (abs(x)=w625:dbl)
    n131 = Greater?(x=w80, y=w79) -> (0:w82:bool)
    n132 = Less?(x=w115, y=10.8) -> (x < y?=w613:bool)
    n133 = Less?(x=w80, y=w78) -> (x < y?=w83:bool)
    n134 = Greater?(x=w17, y=-60.0) -> (0:w572:bool)
    n135 = Greater?(x=w283, y=30.0) -> (0:w300:bool)
    n136 = Greater?(x=w282, y=40.0) -> (0:w291:bool)
    n137 = Greater?(x=w577, y=-60.0) -> (0:w581:bool)
    n138 = Greater?(x=w18, y=-60.0) -> (0:w566:bool)
    n139 = Greater?(x=w542, y=-30.0) -> (0:w559:bool)
    n140 = Greater?(x=w324, y=50.0) -> (0:w341:bool)
    n141 = Greater?(x=w323, y=50.0) -> (0:w332:bool)
    n142 = Greater?(x=w21, y=-30.0) -> (0:w553:bool)
    n143 = Greater?(x=w22, y=-30.0) -> (0:w547:bool)
    n144 = Greater?(x=w521, y=-35.0) -> (0:w539:bool)
    n145 = Greater?(x=w19, y=-35.0) -> (0:w533:bool)
    n146 = Greater?(x=w20, y=-35.0) -> (0:w527:bool)
    n147 = Greater?(x=w157, y=60.0) -> (0:w350:bool)
    n148 = Greater?(x=w284, y=40.0) -> (0:w309:bool)
    n149 = Greater?(x=w382, y=30.0) -> (0:w433:bool)
    n150 = Greater?(x=w325, y=50.0) -> (0:w359:bool)
    n151 = Greater?(x=w381, y=40.0) -> (0:w424:bool)
    n152 = Greater?(x=w380, y=40.0) -> (0:w415:bool)
    n153 = Greater?(x=w103, y=13.2) -> (0:w406:bool)
    n154 = Greater?(x=w379, y=40.0) -> (0:w398:bool)
    n155 = Greater?(x=w378, y=40.0) -> (0:w389:bool)
    n156 = call "Convert from Dynamic Data4"("Dynamic Data Type"=w102) -> ("Scalar"=w94:dbl)  [unwired: 3 in]
    "5s, MGA2805S Out" <- w94
    n157 = Greater?(x=w137, y=w655) -> (0:→"Boolean 8":bool)
    n158 = call "Formula2"("X1"=5000, "X2"=w647, "X3"=28) -> ()  [unwired: 11 in, 2 out]
    n159 = Greater?(x=w23, y=w657) -> (0:w441:bool)
    "Boolean 5" <- w441
    n160 = Greater?(x=w640, y=0.0) -> (0:w630:bool)
    n161 = Greater?(x=w73, y=w72) -> (0:w77:bool)
    n162 = Less?(x=w125, y=w126) -> (x < y?=→"Boolean 75":bool)
    n163 = Less?(x=w121, y=w122) -> (x < y?=→"Boolean 89":bool)
    n164 = Greater?(x=w625, y=0.0) -> (0:w621:bool)
    n165 = Less?(x=w129, y=w130) -> (x < y?=→"Boolean 45":bool)
    n166 = Less?(x=w135, y=w133) -> (x < y?=→"Boolean 18":bool)
    n167 = Or(x=w83, y=w82) -> (x .or. y?=→"Boolean 67":bool)
    n168 = Less?(x=w94, y=4.0) -> (x < y?=w97:bool)
    n169 = Less?(x=w108, y=2.8) -> (x < y?=w104:bool)
    n170 = Greater?(x=w108, y=w107) -> (0:w106:bool)
    n171 = Less?(x=w67, y=2.85) -> (x < y?=w62:bool)
    n172 = Less?(x=w113, y=5.0) -> (x < y?=w110:bool)
    n173 = Less?(x=w73, y=w76) -> (x < y?=w75:bool)
    n174 = And(x=w75, y=w77) -> (x .and. y?=→"Boolean 30":bool)
    n175 = Greater?(x=w67, y=2.0) -> (0:w60:bool)
    n176 = Or(x=w572, y=w571) -> (x .or. y?=w461:bool)
    "Boolean 43" <- w461
    n177 = Or(x=w300, y=w299) -> (x .or. y?=w277:bool)
    "Boolean 85" <- w277
    n178 = Or(x=w291, y=w290) -> (x .or. y?=w274:bool)
    "Boolean 87" <- w274
    n179 = Or(x=w581, y=w580) -> (x .or. y?=w459:bool)
    "Boolean 41" <- w459
    n180 = Or(x=w566, y=w565) -> (x .or. y?=w463:bool)
    "Boolean 47" <- w463
    n181 = Or(x=w559, y=w558) -> (x .or. y?=w465:bool)
    "Boolean 49" <- w465
    n182 = Or(x=w341, y=w340) -> (x .or. y?=w315:bool)
    "Boolean 79" <- w315
    n183 = Or(x=w332, y=w331) -> (x .or. y?=w314:bool)
    "Boolean 81" <- w314
    n184 = Or(x=w553, y=w552) -> (x .or. y?=w467:bool)
    "Boolean 51" <- w467
    n185 = Or(x=w547, y=w546) -> (x .or. y?=w468:bool)
    "Boolean 53" <- w468
    n186 = Or(x=w539, y=w538) -> (x .or. y?=w472:bool)
    "Boolean 55" <- w472
    n187 = Or(x=w533, y=w532) -> (x .or. y?=w474:bool)
    "Boolean 57" <- w474
    n188 = Or(x=w527, y=w526) -> (x .or. y?=w516:bool)
    "Boolean 59" <- w516
    n189 = Or(x=w350, y=w349) -> (x .or. y?=w318:bool)
    "Boolean 77" <- w318
    n190 = Or(x=w309, y=w308) -> (x .or. y?=w278:bool)
    "Boolean 83" <- w278
    n191 = Or(x=w433, y=w432) -> (x .or. y?=w374:bool)
    "Boolean 61" <- w374
    n192 = Or(x=w359, y=w358) -> (x .or. y?=w320:bool)
    "Boolean 73" <- w320
    n193 = Or(x=w424, y=w423) -> (x .or. y?=w373:bool)
    "Boolean 63" <- w373
    n194 = Or(x=w415, y=w414) -> (x .or. y?=w371:bool)
    "Boolean 65" <- w371
    n195 = Or(x=w406, y=w405) -> (x .or. y?=w368:bool)
    n196 = Or(x=w398, y=w397) -> (x .or. y?=w364:bool)
    "Boolean 69" <- w364
    n197 = Or(x=w389, y=w388) -> (x .or. y?=w367:bool)
    "Boolean 71" <- w367
    n198 = Less?(x=w51, y=2.75) -> (x < y?=w53:bool)
    n199 = Greater?(x=w113, y=w112) -> (0:w111:bool)
    n200 = Greater?(x=w115, y=13.2) -> (0:w614:bool)
    n201 = Or(x=w614, y=w613) -> (x .or. y?=w66:bool)
    "Boolean 16" <- w66
    n202 = Greater?(x=w51, y=2.0) -> (0:w54:bool)
    n203 = Less?(x=w40, y=2.75) -> (x < y?=w45:bool)
    n204 = Greater?(x=w40, y=2.0) -> (0:w46:bool)
    n205 = And(x=w106, y=w104) -> (x .and. y?=w105:bool)
    "Boolean 24" <- w105
    n206 = And(x=w62, y=w60) -> (x .and. y?=→"Boolean 33":bool)
    n207 = And(x=w111, y=w110) -> (x .and. y?=→"Boolean 21":bool)
    n208 = And(x=w53, y=w54) -> (x .and. y?=→"Boolean 36":bool)
    n209 = Greater?(x=w94, y=6.0) -> (0:w98:bool)
    n210 = And(x=w45, y=w46) -> (x .and. y?=→"Boolean 39":bool)
    n211 = Greater?(x=w125, y=w126) -> (0:→"Boolean 46":bool)
    n212 = Greater?(x=w121, y=w122) -> (0:→"Boolean 76":bool)
    n213 = Greater?(x=w129, y=w130) -> (0:→"Boolean 19":bool)
    n214 = Greater?(x=w135, y=w133) -> (0:→"Boolean 9":bool)
    n215 = Greater?(x=w80, y=w84) -> (0:w85:bool)
    n216 = Less?(x=w80, y=w79) -> (x < y?=w86:bool)
    n217 = Less?(x=w137, y=w655) -> (x < y?=w443:bool)
    "Boolean 7" <- w443
    n218 = Greater?(x=w142, y=25.0) -> (0:w138:bool)
    n219 = Less?(x=w142, y=27.0) -> (x < y?=w139:bool)
    n220 = Less?(x=w73, y=10.0) -> (x < y?=w601:bool)
    n221 = Or(x=w604, y=w601) -> (x .or. y?=w600:bool)
    "Boolean 29" <- w600
    n222 = Or(x=w98, y=w97) -> (x .or. y?=w99:bool)
    "Boolean 26" <- w99
    n223 = Less?(x=w117, y=27.0) -> (x < y?=w120:bool)
    n224 = Greater?(x=w73, y=10.0) -> (0:w69:bool)
    n225 = Not(x=w461) -> (.not. x?=→"Boolean 44":bool)
    n226 = Not(x=w277) -> (.not. x?=→"Boolean 86":bool)
    n227 = Not(x=w274) -> (.not. x?=→"Boolean 88":bool)
    n228 = Greater?(x=w117, y=25.0) -> (0:w116:bool)
    n229 = Not(x=w459) -> (.not. x?=→"Boolean 42":bool)
    n230 = Not(x=w463) -> (.not. x?=→"Boolean 48":bool)
    n231 = Not(x=w465) -> (.not. x?=→"Boolean 50":bool)
    n232 = Not(x=w315) -> (.not. x?=→"Boolean 80":bool)
    n233 = Not(x=w314) -> (.not. x?=→"Boolean 82":bool)
    n234 = Not(x=w467) -> (.not. x?=→"Boolean 52":bool)
    n235 = Not(x=w468) -> (.not. x?=→"Boolean 54":bool)
    n236 = Not(x=w472) -> (.not. x?=→"Boolean 56":bool)
    n237 = Not(x=w474) -> (.not. x?=→"Boolean 58":bool)
    n238 = Not(x=w516) -> (.not. x?=→"Boolean 60":bool)
    n239 = Not(x=w318) -> (.not. x?=→"Boolean 78":bool)
    n240 = Not(x=w278) -> (.not. x?=→"Boolean 84":bool)
    n241 = Not(x=w374) -> (.not. x?=→"Boolean 62":bool)
    n242 = Not(x=w320) -> (.not. x?=→"Boolean 74":bool)
    n243 = Not(x=w373) -> (.not. x?=→"Boolean 64":bool)
    n244 = Not(x=w371) -> (.not. x?=→"Boolean 66":bool)
    n245 = Not(x=w364) -> (.not. x?=→"Boolean 70":bool)
    n246 = Not(x=w367) -> (.not. x?=→"Boolean 72":bool)
    n247 = And(x=w86, y=w85) -> (x .and. y?=→"Boolean 68":bool)
    n248 = Less?(x=w73, y=w72) -> (x < y?=w70:bool)
    n249 = Less?(x=w26, y=w25) -> (x < y?=w34:bool)
    n250 = And(x=w139, y=w138) -> (x .and. y?=w140:bool)
    "Boolean 11" <- w140
    n251 = Greater?(x=w113, y=5.0) -> (0:w37:bool)
    n252 = Less?(x=w33, y=w32) -> (x < y?=w38:bool)
    n253 = Greater?(x=w108, y=2.8) -> (0:w35:bool)
    n254 = Less?(x=w67, y=2.0) -> (x < y?=→"Boolean 34":bool)
    n255 = And(x=w70, y=w69) -> (x .and. y?=→"Boolean 31":bool)
    n256 = And(x=w120, y=w116) -> (x .and. y?=w119:bool)
    "Boolean 14" <- w119
    n257 = Not(x=w66) -> (.not. x?=→"Boolean 17":bool)
    n258 = Or(x=w35, y=w34) -> (x .or. y?=→"Boolean 25":bool)
    n259 = Or(x=w37, y=w38) -> (x .or. y?=→"Boolean 22":bool)
    n260 = Less?(x=w40, y=2.0) -> (x < y?=→"Boolean 40":bool)
    n261 = Less?(x=w51, y=2.0) -> (x < y?=→"Boolean 37":bool)
    n262 = Equal?(x=w443, y=w442) -> (x = y?=w478:bool)
    n263 = Equal?(x=w441, y=w440) -> (x = y?=w475:bool)
    n264 = Equal?(x=w459, y=w187) -> (x = y?=w493:bool)
    n265 = Equal?(x=w461, y=w460) -> (x = y?=w496:bool)
    n266 = Equal?(x=w277, y=w276) -> (x = y?=w294:bool)
    n267 = Equal?(x=w274, y=w275) -> (x = y?=w285:bool)
    n268 = Equal?(x=w463, y=w462) -> (x = y?=w499:bool)
    n269 = Equal?(x=w468, y=w469) -> (x = y?=w508:bool)
    n270 = Equal?(x=w315, y=w316) -> (x = y?=w335:bool)
    n271 = Equal?(x=w314, y=w313) -> (x = y?=w326:bool)
    n272 = Equal?(x=w472, y=w471) -> (x = y?=w510:bool)
    n273 = Equal?(x=w474, y=w473) -> (x = y?=w513:bool)
    n274 = Equal?(x=w516, y=w517) -> (x = y?=w518:bool)
    n275 = Equal?(x=w318, y=w317) -> (x = y?=w344:bool)
    n276 = Equal?(x=w278, y=w279) -> (x = y?=w303:bool)
    n277 = Equal?(x=w465, y=w464) -> (x = y?=w502:bool)
    n278 = Equal?(x=w374, y=w375) -> (x = y?=w427:bool)
    n279 = Equal?(x=w320, y=w319) -> (x = y?=w353:bool)
    n280 = Or(x=w600, y=w77) -> (x .or. y?=w458:bool)
    n281 = Equal?(x=w467, y=w466) -> (x = y?=w505:bool)
    n282 = Equal?(x=w373, y=w372) -> (x = y?=w418:bool)
    n283 = Equal?(x=w371, y=w370) -> (x = y?=w409:bool)
    n284 = Equal?(x=w368, y=w369) -> (x = y?=w401:bool)
    n285 = Equal?(x=w364, y=w365) -> (x = y?=w392:bool)
    n286 = Equal?(x=w367, y=w366) -> (x = y?=w383:bool)
    n287 = Not(x=w99) -> (.not. x?=→"Boolean 27":bool)
    n288 = Not(x=w478) -> (.not. x?=w479:bool)
    n289 = Not(x=w475) -> (.not. x?=w476:bool)
    n290 = Not(x=w493) -> (.not. x?=w494:bool)
    n291 = call "Formula"("X1"="A", "X2"="B", "X3"="C") -> ("Result"=w649:dynamicdata)  [unwired: 11 in, 1 out]
    n292 = Less?(x=w142, y=25.0) -> (x < y?=w629:bool)
    n293 = And(x=w630, y=w629) -> (x .and. y?=w626:bool)
    "Boolean 10" <- w626
    n294 = Not(x=w496) -> (.not. x?=w497:bool)
    n295 = Not(x=w294) -> (.not. x?=w295:bool)
    n296 = Not(x=w285) -> (.not. x?=w286:bool)
    n297 = Less?(x=w117, y=25.0) -> (x < y?=w620:bool)
    n298 = And(x=w621, y=w620) -> (x .and. y?=w617:bool)
    "Boolean 13" <- w617
    n299 = Not(x=w499) -> (.not. x?=w500:bool)
    n300 = Not(x=w508) -> (.not. x?=w509:bool)
    n301 = Not(x=w335) -> (.not. x?=w336:bool)
    n302 = Not(x=w326) -> (.not. x?=w327:bool)
    n303 = Not(x=w510) -> (.not. x?=w511:bool)
    n304 = Not(x=w513) -> (.not. x?=w514:bool)
    n305 = Not(x=w518) -> (.not. x?=w519:bool)
    n306 = Not(x=w344) -> (.not. x?=w345:bool)
    n307 = Not(x=w303) -> (.not. x?=w304:bool)
    n308 = Not(x=w502) -> (.not. x?=w503:bool)
    n309 = Not(x=w427) -> (.not. x?=w428:bool)
    n310 = Not(x=w353) -> (.not. x?=w354:bool)
    n311 = Not(x=w505) -> (.not. x?=w506:bool)
    n312 = Not(x=w418) -> (.not. x?=w419:bool)
    n313 = Not(x=w409) -> (.not. x?=w410:bool)
    n314 = Not(x=w401) -> (.not. x?=w402:bool)
    n315 = Not(x=w392) -> (.not. x?=w393:bool)
    n316 = Not(x=w383) -> (.not. x?=w384:bool)
    n317 = Greater?(x=w80, y=w78) -> (0:w89:bool)
    n318 = Less?(x=w80, y=w84) -> (x < y?=w90:bool)
    n319 = And(x=w443, y=w479) -> (x .and. y?=w480:bool)
    n320 = case shown="True" w480 {
      frame False {
      }
      frame True {
        n321 = call <vilib>:"Beep.vi"() -> ()  [unwired: 12 in]
      }
    }
    n322 = And(x=w441, y=w476) -> (x .and. y?=w477:bool)
    n323 = case shown="True" w477 {
      frame False {
      }
      frame True {
        n324 = call <vilib>:"Beep.vi"() -> ()  [unwired: 12 in]
      }
    }
    n325 = Or(x=w31, y=w110) -> (x .or. y?=w454:bool)
    n326 = And(x=w459, y=w494) -> (x .and. y?=w495:bool)
    n327 = case shown="True" w495 {
      frame False {
      }
      frame True {
        n328 = call <vilib>:"Beep.vi"() -> ()  [unwired: 12 in]
      }
    }
    n329 = And(x=w461, y=w497) -> (x .and. y?=w498:bool)
    n330 = case shown="True" w498 {
      frame False {
      }
      frame True {
        n331 = call <vilib>:"Beep.vi"() -> ()  [unwired: 12 in]
      }
    }
    n332 = And(x=w277, y=w295) -> (x .and. y?=w296:bool)
    n333 = case shown="True" w296 {
      frame False {
      }
      frame True {
        n334 = call <vilib>:"Beep.vi"() -> ()  [unwired: 12 in]
      }
    }
    n335 = And(x=w274, y=w286) -> (x .and. y?=w287:bool)
    n336 = case shown="True" w287 {
      frame False {
      }
      frame True {
        n337 = call <vilib>:"Beep.vi"() -> ()  [unwired: 12 in]
      }
    }
    n338 = And(x=w463, y=w500) -> (x .and. y?=w501:bool)
    n339 = case shown="True" w501 {
      frame False {
      }
      frame True {
        n340 = call <vilib>:"Beep.vi"() -> ()  [unwired: 12 in]
      }
    }
    n341 = And(x=w468, y=w509) -> (x .and. y?=w470:bool)
    n342 = case shown="True" w470 {
      frame False {
      }
      frame True {
        n343 = call <vilib>:"Beep.vi"() -> ()  [unwired: 12 in]
      }
    }
    n344 = And(x=w315, y=w336) -> (x .and. y?=w337:bool)
    n345 = case shown="True" w337 {
      frame False {
      }
      frame True {
        n346 = call <vilib>:"Beep.vi"() -> ()  [unwired: 12 in]
      }
    }
    n347 = And(x=w314, y=w327) -> (x .and. y?=w328:bool)
    n348 = case shown="True" w328 {
      frame False {
      }
      frame True {
        n349 = call <vilib>:"Beep.vi"() -> ()  [unwired: 12 in]
      }
    }
    n350 = And(x=w472, y=w511) -> (x .and. y?=w512:bool)
    n351 = case shown="True" w512 {
      frame False {
      }
      frame True {
        n352 = call <vilib>:"Beep.vi"() -> ()  [unwired: 12 in]
      }
    }
    n353 = And(x=w474, y=w514) -> (x .and. y?=w515:bool)
    n354 = case shown="True" w515 {
      frame False {
      }
      frame True {
        n355 = call <vilib>:"Beep.vi"() -> ()  [unwired: 12 in]
      }
    }
    n356 = And(x=w516, y=w519) -> (x .and. y?=w520:bool)
    n357 = case shown="True" w520 {
      frame False {
      }
      frame True {
        n358 = call <vilib>:"Beep.vi"() -> ()  [unwired: 12 in]
      }
    }
    n359 = And(x=w318, y=w345) -> (x .and. y?=w346:bool)
    n360 = case shown="True" w346 {
      frame False {
      }
      frame True {
        n361 = call <vilib>:"Beep.vi"() -> ()  [unwired: 12 in]
      }
    }
    n362 = And(x=w278, y=w304) -> (x .and. y?=w305:bool)
    n363 = case shown="True" w305 {
      frame False {
      }
      frame True {
        n364 = call <vilib>:"Beep.vi"() -> ()  [unwired: 12 in]
      }
    }
    n365 = And(x=w465, y=w503) -> (x .and. y?=w504:bool)
    n366 = case shown="True" w504 {
      frame False {
      }
      frame True {
        n367 = call <vilib>:"Beep.vi"() -> ()  [unwired: 12 in]
      }
    }
    n368 = And(x=w374, y=w428) -> (x .and. y?=w429:bool)
    n369 = case shown="True" w429 {
      frame False {
      }
      frame True {
        n370 = call <vilib>:"Beep.vi"() -> ()  [unwired: 12 in]
      }
    }
    n371 = And(x=w320, y=w354) -> (x .and. y?=w355:bool)
    n372 = case shown="True" w355 {
      frame False {
      }
      frame True {
        n373 = call <vilib>:"Beep.vi"() -> ()  [unwired: 12 in]
      }
    }
    n374 = And(x=w467, y=w506) -> (x .and. y?=w507:bool)
    n375 = case shown="True" w507 {
      frame False {
      }
      frame True {
        n376 = call <vilib>:"Beep.vi"() -> ()  [unwired: 12 in]
      }
    }
    n377 = And(x=w373, y=w419) -> (x .and. y?=w420:bool)
    n378 = case shown="True" w420 {
      frame False {
      }
      frame True {
        n379 = call <vilib>:"Beep.vi"() -> ()  [unwired: 12 in]
      }
    }
    n380 = And(x=w371, y=w410) -> (x .and. y?=w411:bool)
    n381 = case shown="True" w411 {
      frame False {
      }
      frame True {
        n382 = call <vilib>:"Beep.vi"() -> ()  [unwired: 12 in]
      }
    }
    n383 = And(x=w368, y=w402) -> (x .and. y?=w403:bool)
    n384 = case shown="True" w403 {
      frame False {
      }
      frame True {
        n385 = call <vilib>:"Beep.vi"() -> ()  [unwired: 12 in]
      }
    }
    n386 = And(x=w364, y=w393) -> (x .and. y?=w394:bool)
    n387 = case shown="True" w394 {
      frame False {
      }
      frame True {
        n388 = call <vilib>:"Beep.vi"() -> ()  [unwired: 12 in]
      }
    }
    n389 = And(x=w367, y=w384) -> (x .and. y?=w385:bool)
    n390 = case shown="True" w385 {
      frame False {
      }
      frame True {
        n391 = call <vilib>:"Beep.vi"() -> ()  [unwired: 12 in]
      }
    }
    n392 = And(x=w90, y=w89) -> (x .and. y?=→"Boolean 90":bool)
    n393 = Or(x=w28, y=w105) -> (x .or. y?=w456:bool)
    n394 = Greater?(x=w142, y=27.0) -> (0:→"Boolean 12":bool)
    n395 = Greater?(x=w117, y=27.0) -> (0:→"Boolean 15":bool)
    n396 = call "Convert from Dynamic Data"("Dynamic Data Type"=w649) -> ("Array"=w648:dbl[])  [unwired: 3 in]
    n397 = Or(x=w626, y=w140) -> (x .or. y?=w92:bool)
    n398 = Or(x=w617, y=w119) -> (x .or. y?=w445:bool)
    n399 = Build Array(w137, w129) -> (w641:dbl[])
    n400 = Build Array(w67, w51, w40) -> (w592:dbl[])
    n401 = Build Array(w23, w125) -> (w636:dbl[])
    n402 = Build Array(w135, w121) -> (w633:dbl[])
    n403 = Build Array(w542, w22, w21) -> (w147:dbl[])
    n404 = Build Array (concatenate)(w651, w648) -> (w650:dbl[][])
    n405 = Build Array (concatenate)(w610, w113) -> (w438:dbl[])
    n406 = Build Array (concatenate)(w606, w108) -> (w437:dbl[])
    n407 = Build Array(w577, w18, w17) -> (w576:dbl[])
    n408 = Build Array (concatenate)(w653, w641) -> (w652:dbl[][])
    n409 = Build Array (concatenate)(w635, w636) -> (w634:dbl[][])
    n410 = Build Array (concatenate)(w632, w633) -> (w631:dbl[][])
    n411 = Build Array(w325, w157, w324, w323) -> (w321:dbl[])
    n412 = Equal?(x=w458, y=w457) -> (x = y?=w490:bool)
    n413 = Equal?(x=w454, y=w453) -> (x = y?=w484:bool)
    n414 = Equal?(x=w456, y=w455) -> (x = y?=w487:bool)
    n415 = Build Array(w521, w20, w19) -> (w523:dbl[])
    n416 = Build Array(w382, w381, w380, w379, w378) -> (w377:dbl[])
    n417 = Build Array(w284, w283, w282) -> (w281:dbl[])
    n418 = Not(x=w490) -> (.not. x?=w491:bool)
    n419 = Not(x=w484) -> (.not. x?=w485:bool)
    n420 = Not(x=w487) -> (.not. x?=w488:bool)
    n421 = Build Array (concatenate)(w186, w73) -> (w436:dbl[])
    n422 = Build Array (concatenate)(w593, w592) -> (w591:dbl[][])
    n423 = Build Array (concatenate)(w280, w281) -> (w273:dbl[][])
    n424 = Build Array (concatenate)(w575, w576) -> (w562:dbl[][])
    n425 = Build Array (concatenate)(w543, w147) -> (w148:dbl[][])
    n426 = And(x=w458, y=w491) -> (x .and. y?=w492:bool)
    n427 = case shown="True" w492 {
      frame False {
      }
      frame True {
        n428 = call <vilib>:"Beep.vi"() -> ()  [unwired: 12 in]
      }
    }
    n429 = Equal?(x=w66, y=w180) -> (x = y?=w481:bool)
    n430 = And(x=w454, y=w485) -> (x .and. y?=w486:bool)
    n431 = case shown="True" w486 {
      frame False {
      }
      frame True {
        n432 = call <vilib>:"Beep.vi"() -> ()  [unwired: 12 in]
      }
    }
    n433 = Build Array (concatenate)(w522, w523) -> (w363:dbl[][])
    n434 = And(x=w456, y=w488) -> (x .and. y?=w489:bool)
    n435 = case shown="True" w489 {
      frame False {
      }
      frame True {
        n436 = call <vilib>:"Beep.vi"() -> ()  [unwired: 12 in]
      }
    }
    n437 = Build Array (concatenate)(w322, w321) -> (w312:dbl[][])
    n438 = Build Array (concatenate)(w376, w377) -> (w362:dbl[][])
    n439 = Not(x=w481) -> (.not. x?=w482:bool)
    n440 = Equal?(x=w92, y=w446) -> (x = y?=w447:bool)
    n441 = Equal?(x=w445, y=w444) -> (x = y?=w450:bool)
    n442 = And(x=w66, y=w482) -> (x .and. y?=w483:bool)
    n443 = case shown="True" w483 {
      frame False {
      }
      frame True {
        n444 = call <vilib>:"Beep.vi"() -> ()  [unwired: 12 in]
      }
    }
    n445 = Not(x=w447) -> (.not. x?=w448:bool)
    n446 = Not(x=w450) -> (.not. x?=w451:bool)
    n447 = And(x=w92, y=w448) -> (x .and. y?=w449:bool)
    n448 = case shown="True" w449 {
      frame False {
      }
      frame True {
        n449 = call <vilib>:"Beep.vi"() -> ()  [unwired: 12 in]
      }
    }
    n450 = And(x=w445, y=w451) -> (x .and. y?=w452:bool)
    n451 = case shown="True" w452 {
      frame False {
      }
      frame True {
        n452 = call <vilib>:"Beep.vi"() -> ()  [unwired: 12 in]
      }
    }
  }
  "Iout" <- w16
  "I12d+" <- w15
  "I5s" <- w14
  "TEC Currents" <- w13
  "Cold Fingers" <- w12
  "Back Plates" <- w11
  "CONT" <- w10
  "PCU" <- w9
  "COMP" <- w8
  "Reservoir" <- w7
  "0 Order TECs" <- w6
  "-1 Order TECs" <- w5
  "+1 Order TECs" <- w4
  n453 = invoke on="Power" class="SubPanel" method="Remove VI"() -> ()  [unwired: 3 in, 3 out]
  n454 = while {
    tunnel: [w715] -> w3
    tunnel: [w714] -> w1
    tunnel: [w713] -> w2
    stop <- w728 stop-if-true
    n455 = control-ref of="Output Array"() -> (w727:refnum<vi>)
    n456 = local read "stop 2"() -> (w728:bool)
    n457 = call "MOSES Background 4_v8.vi"("Array Input"=w727) -> ("PSU"=w714:dbl[], "Values to Output"=w726:T5, "Power Supply Filter Input"=w715:dbl[], "ROE"=w713:dbl[])  [unwired: 1 in]
    n458 = Unbundle By Name(w726) -> ("T5V, Thermal 5V power voltage"=→"Thermal 5V power":dbl, "S28V, Shutter 28V power voltage"=→"Shutter 28V power":dbl, "HAFV, H-alpha filter voltage"=→"H-alpha filter":dbl, "HACV, H-alpha camera voltage"=→"H-alpha camera":dbl, "Ipf12+, Premod filter positive 12V input current"=→"Premod filter positive 12V input":dbl, "I_pf5, Premod filter 5V input current"=→"Premod filter 5V input":dbl, "S28I, Shutter 28V power current"=→"Shutter 28V power":dbl, "HAFI, H-alpha filter current"=→"H-alpha filter":dbl, "ROE_PSV, ROE power supply input voltage"=→"ROE power supply input":dbl, "ROE_PSI, ROE power supply input current"=→"ROE power supply input":dbl)  [unwired: 9 out]
  }
  "Power Supply Filter Input" <- w3
  "PSU" <- w1
  "ROE" <- w2
